vi "FTW-File-ListDirectories.vi"(0 "Directories":path[](array[path]), 5 "Matching Filename Pattern":string, 7 "Matching Directory Pattern":string, 9 "Treat LLBs as Folders?":bool=TRUE, 11 "error in":errorcluster) -> (6 "Matching Filepaths":path[](array[path]), 8 "Num Files Found":i32, 15 "error out":errorcluster)   [LabVIEW 2015]
uses:
  regex/FTW-Regex.vi
  regex/FTW-Regex-Execute.vi
  error/FTW-ERR-ThrowGenericError.vi
  error/FTW-ERR-ThrowError.vi
  error/FTW-ERR-CallChain.vi
  error/FTW-ERR-NoErrorConstant.vi
  string/FTW-STR-ReplaceWhitespace.vi
  string/FTW-STR-Array-Delimit.vi
  regex/FTW-Regex-ReplaceAll.vi
  regex/FTW-Regex-Construct.vi
  lib/FTW-KernelFilepath.vi
  regex/FTW-Regex-Destroy.vi
panel:
  # "Inputs"
  # "Outputs"
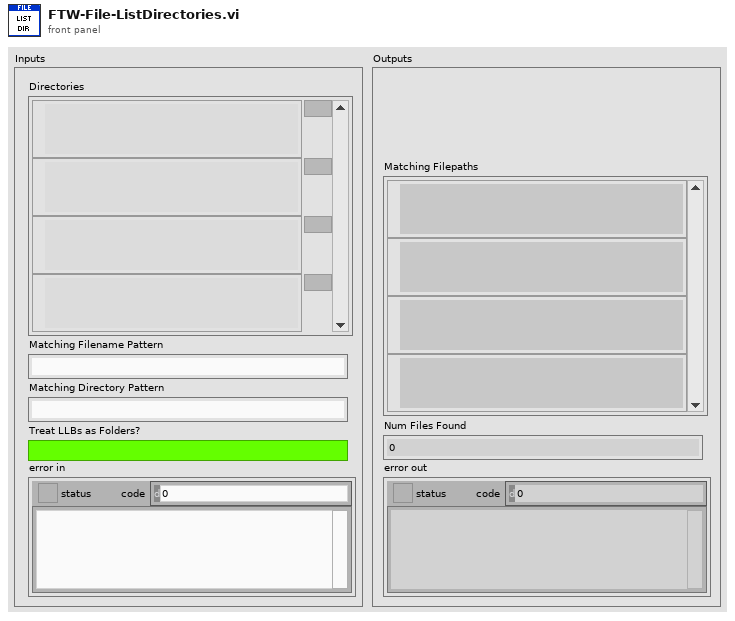
[diagram p1: front panel]
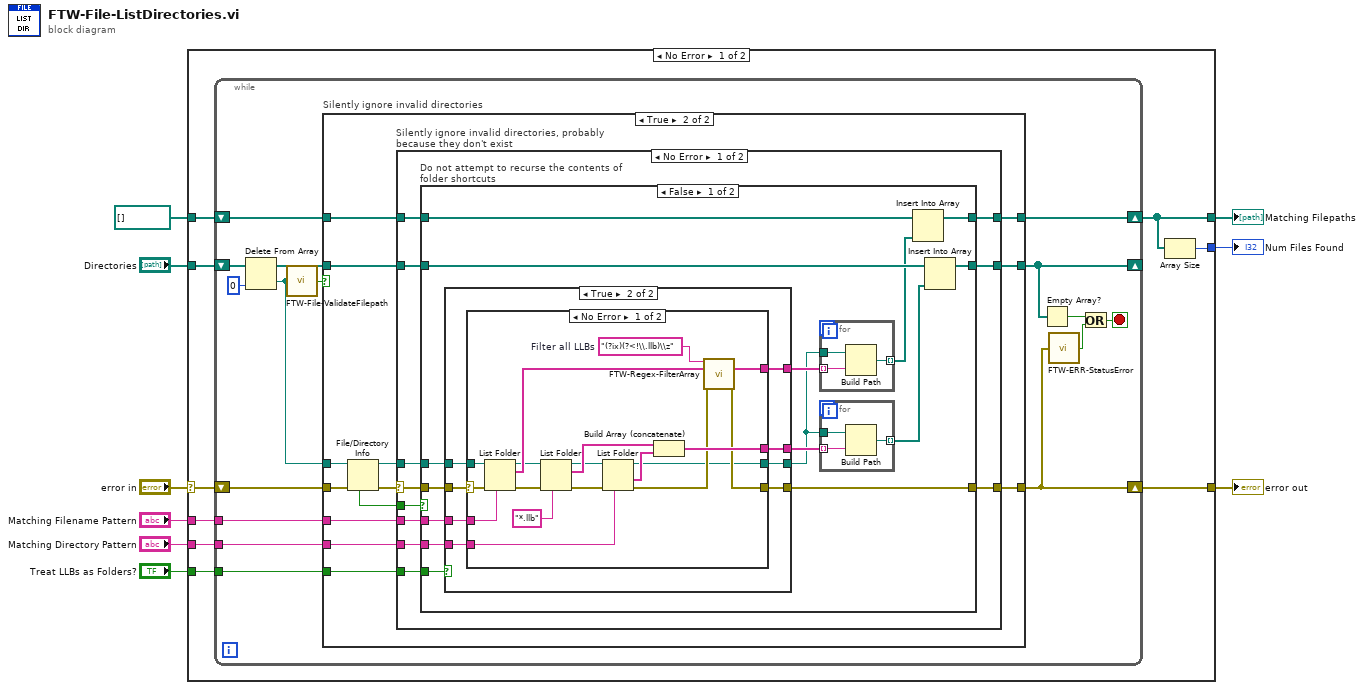
[diagram p0: block diagram]
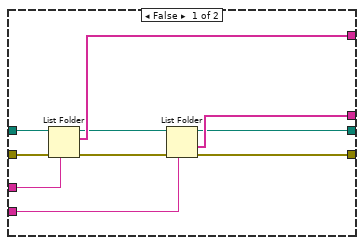
[diagram p3: hidden frame]
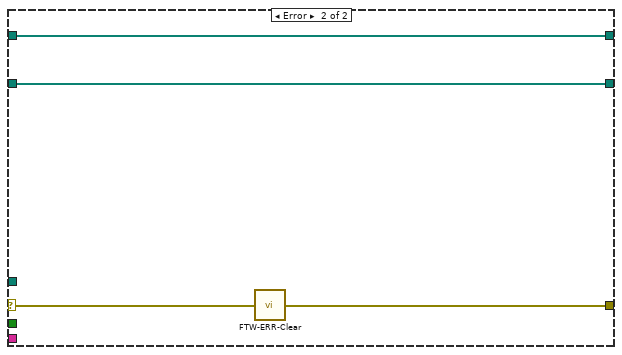
[diagram p6: hidden frame]
diagram:
  n1 = case shown="No Error" "error in" {
    selector: "error in" -> [w15 w129]
    tunnel: [w11 w128] -> w9
    tunnel: [w16 w129] -> w5
    tunnel: "Treat LLBs as Folders?" -> [w18 _]
    tunnel: "Matching Filename Pattern" -> [w17 _]
    tunnel: "Matching Directory Pattern" -> [w14 _]
    tunnel: path[] [] -> [w13 w128]
    tunnel: [w12 _] -> w2
    tunnel: "Directories" -> [w10 _]
    frame No Error {
      n2 = while {
        shift-left: w13 -> [w32]
        shift-right: [w34] -> w11
        shift-left: w10 -> [w33]
        shift-right: [w29] -> _
        shift-right: [w22] -> w16
        shift-left: w15 -> [w27]
        tunnel: w18 -> [w31]
        tunnel: w17 -> [w30]
        tunnel: w14 -> [w25]
        stop <- w19 stop-if-true
        n3 = Delete From Array(array=w33, index=0) -> (deleted portion=w24:path, array with subset deleted=w26:path[])  [unwired: 1 in]
        n4 = call "FTW-File-ValidateFilepath.vi"("Filepath"=w24) -> ("Valid?"=w23:bool)
        n5 = case "Silently ignore invalid directories" shown="True" w23 {
          tunnel: [w37 w38] -> w34
          tunnel: w32 -> [w37 w39]
          tunnel: w31 -> [_ w50]
          tunnel: w30 -> [_ w49]
          tunnel: [w36 w40] -> w29
          tunnel: [w35 w48] -> w22
          tunnel: w24 -> [_ w47]
          tunnel: w27 -> [w35 w44]
          tunnel: w26 -> [w36 w41]
          tunnel: w25 -> [_ w43]
          frame False {
          }
          frame True {
            n6 = File/Directory Info(path=w47, error in=w44) -> (path out=w46:path, error out=w42:errorcluster, shortcut=w45:bool)  [unwired: 4 out]
            n7 = case "Silently ignore invalid directories, probably because they don't exist" shown="No Error" w42 {
              selector: w42 -> [w55 w125]
              tunnel: w50 -> [w61 _]
              tunnel: w49 -> [w60 _]
              tunnel: [w59 w124] -> w48
              tunnel: w46 -> [w58 _]
              tunnel: w45 -> [w57 _]
              tunnel: w43 -> [w56 _]
              tunnel: w41 -> [w54 w126]
              tunnel: [w53 w126] -> w40
              tunnel: w39 -> [w52 w127]
              tunnel: [w51 w127] -> w38
              frame No Error {
                n8 = case "Do not attempt to recurse the contents of folder shortcuts" shown="False" w57 {
                  tunnel: [w76 w123] -> w59
                  tunnel: w61 -> [w75 _]
                  tunnel: w60 -> [w74 _]
                  tunnel: w55 -> [w73 w123]
                  tunnel: w58 -> [w72 _]
                  tunnel: w56 -> [w71 _]
                  tunnel: w54 -> [w66 w122]
                  tunnel: [w65 w122] -> w53
                  tunnel: w52 -> [w64 w121]
                  tunnel: [w62 w121] -> w51
                  frame False {
                    n9 = case shown="True" w75 {
                      tunnel: [w92 w97] -> w70
                      tunnel: [w86 w98] -> w69
                      tunnel: w72 -> [w91 w94]
                      tunnel: [w83 w93] -> w68
                      tunnel: [w87 w99] -> w76
                      tunnel: w73 -> [w90 w100]
                      tunnel: w74 -> [w89 w96]
                      tunnel: w71 -> [w84 w95]
                      frame False {
                        n10 = List Folder(path=w91, pattern=w89, error in=w90) -> (path out=w85:path, filenames=w92:string[], error out=w88:errorcluster)  [unwired: 2 out]
                        n11 = List Folder(path=w85, pattern=w84, error in=w88) -> (path out=w83:path, folder names=w86:string[], error out=w87:errorcluster)  [unwired: 2 out]
                      }
                      frame True {
                        n12 = case shown="No Error" w100 {
                          selector: w100 -> [w117 w120]
                          tunnel: [w107 _] -> w97
                          tunnel: w94 -> [w118 w119]
                          tunnel: [w105 w120] -> w99
                          tunnel: [w110 _] -> w98
                          tunnel: w96 -> [w116 _]
                          tunnel: w95 -> [w103 _]
                          tunnel: [w102 w119] -> w93
                          frame No Error {
                            w104 = "(?ix)(?<!\\.llb)\\z"  # Filter all LLBs
                            n13 = List Folder(path=w118, pattern=w116, error in=w117) -> (path out=w101:path, filenames=w106:string[], error out=w115:errorcluster)  [unwired: 2 out]
                            n14 = List Folder(path=w101, pattern="*.llb", error in=w115) -> (path out=w109:path, filenames=w111:string[], error out=w113:errorcluster)  [unwired: 2 out]
                            n15 = List Folder(path=w109, pattern=w103, error in=w113) -> (path out=w102:path, folder names=w112:string[], error out=w108:errorcluster)  [unwired: 2 out]
                            n16 = Build Array (concatenate)(w111, w112) -> (w110:string[])
                            n17 = call "FTW-Regex-FilterArray.vi"("Regex Filter"=w104, "Input Array"=w106, "error in"=w108) -> ("Matching Items"=w107:string[], "error out"=w105:errorcluster)  [unwired: 10 in, 1 out]
                          }
                          frame Error {
                          }
                        }
                      }
                    }
                    n18 = for {
                      tunnel: w68 -> [w82]
                      tunnel: [w81] -> w63 mode=indexing
                      tunnel: w70 -> [w80] mode=indexing
                      n19 = Build Path(base path=w82, name or relative path=w80) -> (appended path=w81:path)
                    }
                    n20 = for {
                      tunnel: w68 -> [w79]
                      tunnel: [w78] -> w67 mode=indexing
                      tunnel: w69 -> [w77] mode=indexing
                      n21 = Build Path(base path=w79, name or relative path=w77) -> (appended path=w78:path)
                    }
                    n22 = Insert Into Array(array=w64, new element=w63) -> (w62:path[])  [unwired: 1 in]
                    n23 = Insert Into Array(array=w66, new element=w67) -> (w65:path[])  [unwired: 1 in]
                  }
                  frame True {
                  }
                }
              }
              frame Error {
                n24 = call "FTW-ERR-Clear.vi"("error to snuff"=w125) -> ("no error"=w124:errorcluster)
              }
            }
          }
        }
        n25 = Empty Array?(array=w29) -> (empty?=w21:bool)
        n26 = call "FTW-ERR-StatusError.vi"("error to check"=w22) -> ("Error?"=w20:bool)
        n27 = Or(x=w21, y=w20) -> (x .or. y?=w19:bool)
      }
      n28 = Array Size(array=w11) -> (size(s)=w12:i32)
    }
    frame Error {
    }
  }
  "Matching Filepaths" <- w9
  "error out" <- w5
  "Num Files Found" <- w2
